vi "MotorMoveIRL.vi"(11 "Rbt Cmd":string) -> ()   [LabVIEW 2019]
uses:
  <vilib>/myRIO/Instrument Drivers/Onboard IO/DIO/typedefs/DIO Reference.ctl
  <vilib>/myRIO/Common/Instrument Driver Framework/Utilities/typedefs/myRIO Generic Hardware Reference.ctl
  <vilib>/myRIO/Common/Instrument Driver Framework/Utilities/typedefs/Hardware Version Enum.ctl
  <vilib>/myRIO/Common/Instrument Driver Framework/Utilities/typedefs/myRIO v1.0 Reference.ctl
  <vilib>/myRIO/Common/Instrument Driver Framework/Utilities/typedefs/Generic FPGA Reference.ctl
  <vilib>/myRIO/Common/Instrument Driver Framework/myRIO v1.0/DIO/typedefs/DIO Channels List.ctl
  <vilib>/myRIO/Common/Instrument Driver Framework/myRIO v1.0/DIO/typedefs/DIO Channels Enum.ctl
  <vilib>/userDefined/High Color/nirio_resource_hc.ctl
  <vilib>/myRIO/Instrument Drivers/Onboard IO/AO/typedefs/AO Reference.ctl
  <vilib>/myRIO/Common/Instrument Driver Framework/myRIO v1.0/AO/typedefs/AO Channels List.ctl
  <vilib>/myRIO/Common/Instrument Driver Framework/myRIO v1.0/AO/typedefs/AO Channels Enum.ctl
  <vilib>/myRIO/Common/Instrument Driver Framework/Utilities/typedefs/Analog Scaling Constants List.ctl
  <vilib>/myRIO/Common/Instrument Driver Framework/Utilities/typedefs/Analog Scaling Constants.ctl
  <vilib>/myRIO/Common/Instrument Driver Framework/myRIO v1.0/Encoder/typedefs/Encoder Signal Mode.ctl
  <vilib>/myRIO/Instrument Drivers/Onboard IO/Encoder/typedefs/Encoder Reference.ctl
  <vilib>/myRIO/Common/Instrument Driver Framework/myRIO v1.0/Encoder/typedefs/Encoder Channels Enum.ctl
  <vilib>/myRIO/Common/Instrument Driver Framework/myRIO v1.0/Encoder/typedefs/Encoder Configuration v1.0.ctl
  <vilib>/myRIO/Common/Instrument Driver Framework/Utilities/vis/Is FPGA Ref Available.vi
  <vilib>/myRIO/Common/Instrument Driver Framework/myRIO v1.0/DIO/vis/myRIO v1.1 Open DIO.vi
  <vilib>/myRIO/Instrument Drivers/Onboard IO/DIO/vis/Write.vi
  <vilib>/myRIO/Common/Instrument Driver Framework/myRIO v1.0/AO/vis/myRIO v1.1 Open AO.vi
  <vilib>/myRIO/Instrument Drivers/Onboard IO/AO/vis/Write.vi
  <vilib>/myRIO/Common/Instrument Driver Framework/myRIO v1.0/Encoder/vis/myRIO v1.1 Open Encoder.vi
  <vilib>/myRIO/Instrument Drivers/Onboard IO/Encoder/vis/Read.vi
  <vilib>/myRIO/Common/Instrument Driver Framework/Utilities/vis/Validate Channels.vi
  <vilib>/myRIO/Common/Instrument Driver Framework/myRIO v1.0/DIO/vis/myRIO v1.0 Reserve DIO.vi
  <vilib>/myRIO/Common/Instrument Driver Framework/myRIO v1.0/AO/vis/myRIO v1.0 Reserve AO.vi
  <vilib>/myRIO/Common/Instrument Driver Framework/myRIO v1.0/Encoder/vis/myRIO v1.0 Reserve Encoder.vi
  <vilib>/myRIO/Common/Instrument Driver Framework/myRIO v1.0/Resource Manager/vis/myRIO v1.0 Reserve Channel List.vi
  <vilib>/myRIO/Common/Instrument Driver Framework/myRIO v1.0/DIO/vis/myRIO v1.0 Build MUX Configuration DIO.vi
  <vilib>/myRIO/Common/Instrument Driver Framework/myRIO v1.0/AO/vis/myRIO v1.0 Build MUX Configuration AO.vi
  <vilib>/myRIO/Common/Instrument Driver Framework/myRIO v1.0/Encoder/vis/myRIO v1.0 Build MUX Configuration Encoder.vi
  <vilib>/myRIO/Common/Instrument Driver Framework/myRIO v1.0/Resource Manager/vis/myRIO v1.0 Reserve Channel.vi
  <vilib>/myRIO/Common/Instrument Driver Framework/myRIO v1.0/Resource Manager/vis/myRIO v1.0 Unreserve Channel.vi
  <vilib>/myRIO/Common/Instrument Driver Framework/myRIO v1.0/Resource Manager/vis/myRIO v1.0 Create Configuration List.vi
  <vilib>/myRIO/Common/Instrument Driver Framework/myRIO v1.0/Resource Manager/vis/myRIO v1.0 Build Mutex Name.vi
  <vilib>/Utility/VariantDataType/GetNumericInfo.vi
  <vilib>/Utility/error.llb/Error Cluster From Error Code.vi
  <vilib>/myRIO/Common/Instrument Driver Framework/myRIO v1.0/myRIO v1.1 Open.vi
  <vilib>/myRIO/Common/Instrument Driver Framework/Utilities/vis/IO Manager.vi
  <vilib>/myRIO/Common/Instrument Driver Framework/Utilities/vis/Configuration Manager.vi
  <vilib>/myRIO/Common/Instrument Driver Framework/myRIO v1.0/Resource Manager/vis/myRIO v1.0 Configure IO.vi
  <vilib>/myRIO/Common/Instrument Driver Framework/myRIO v1.0/myRIO v1.0 Close.vi
  <vilib>/myRIO/Common/Instrument Driver Framework/myRIO v1.0/DIO/vis/myRIO v1.0 Write DIO.vi
  <vilib>/myRIO/Common/Instrument Driver Framework/myRIO v1.0/AO/vis/myRIO v1.0 Get Scaling Constants AO.vi
  <vilib>/myRIO/Common/Instrument Driver Framework/myRIO v1.0/AO/vis/myRIO v1.0 Write AO.vi
  <vilib>/myRIO/Common/Instrument Driver Framework/myRIO v1.0/Encoder/vis/myRIO v1.0 Configure Encoder.vi
  <vilib>/myRIO/Common/Instrument Driver Framework/myRIO v1.0/Encoder/vis/myRIO v1.0 Read Encoder.vi
  <vilib>/myRIO/Express VI/Onboard IO/DO/DO Express VI.xnode
  <vilib>/myRIO/Instrument Drivers/Onboard IO/DIO/vis/myRIO DIO Open.xnode
  <vilib>/myRIO/Express VI/Onboard IO/AO/AO Express VI.xnode
  <vilib>/myRIO/Instrument Drivers/Onboard IO/AO/vis/myRIO AO Open.xnode
  <vilib>/myRIO/Express VI/Onboard IO/Encoder/Encoder Express VI.xnode
  <vilib>/myRIO/Instrument Drivers/Onboard IO/Encoder/vis/myRIO Encoder Open.xnode
  <vilib>/myRIO/Common/Instrument Driver Framework/myRIO v1.0/Encoder/typedefs/Encoder Count Direction Enum.ctl
  <vilib>/myRIO/Instrument Drivers/Onboard IO/Encoder/Encoder.lvlib
  <vilib>/myRIO/Instrument Drivers/Onboard IO/DIO/DIO.lvlib
  <vilib>/myRIO/Instrument Drivers/Onboard IO/AO/AO.lvlib
panel:
  out "Enco D":i32
  out "Enco U":i32
  out "Enco B":i32
  out "Enco R (2)":i32
  out "Enco L (1)":i32
  out "Enco F":i32
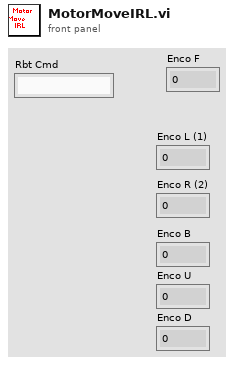
[diagram p1: front panel]
types:
  T1 = typedef "AO.lvlib/AO Reference.ctl" = cluster{"myRIO Reference":T2, "AO Channel List":T6, "AO Scaling Constant List":T8}
  T2 = typedef "myRIO Generic Hardware Reference.ctl" = cluster{"myRIO Model":T3, "myRIO Hardware Reference":T4}
  T3 = typedef "Hardware Version Enum.ctl" = enum16{"Unknown", "myRIO-1900", "myRIO-1950", "roboRIO", "NI ELVIS RIO CM", "ELVIS III"}
  T4 = typedef "myRIO v1.0 Reference.ctl" = cluster{"Generic FPGA Reference":T5, "Allow multiple opens":bool}
  T5 = typedef "Generic FPGA Reference.ctl" = refnum<k20>
  T6 = typedef "AO Channels List.ctl" = T7[]
  T7 = typedef "AO Channels Enum.ctl" = enum16{"Not Connected", "AudioOut/Left", "AudioOut/Right", "C/AO0", "C/AO1", "A/AO0", "A/AO1", "B/AO0", "B/AO1"}
  T8 = typedef "Analog Scaling Constants List.ctl" = T9[]
  T9 = typedef "Analog Scaling Constants.ctl" = cluster{"LSB Weight (Volts)":dbl, "Offset (Volts)":dbl, "Signed?":bool}
  T10 = typedef "nirio_resource_hc.ctl" = tag
  T11 = typedef "Encoder.lvlib/Encoder Reference.ctl" = cluster{"myRIO Reference":T2, "Encoder Channels Enum":T12}
  T12 = typedef "Encoder Channels Enum.ctl" = enum16{"Not Connected", "C/ENC0", "C/ENC1", "A/ENC", "A/ENC0", "A/ENC1", "A/ENC2", "A/ENC3", "A/ENC4", "A/ENC5", "A/ENC6", "A/ENC7", "A/ENC8", "A/ENC9", "B/ENC", "B/ENC0", "B/ENC1", "B/ENC2", "B/ENC3", "B/ENC4", "B/ENC5", "B/ENC6", "B/ENC7", "B/ENC8", "B/ENC9", "DIO/ENC0", "DIO/ENC1", "DIO/ENC2", "DIO/ENC3", "DIO/ENC4"}
  T13 = typedef "Encoder Signal Mode.ctl" = enum16{"Quadrature phase signal", "Step and direction signal"}
  T14 = typedef "DIO.lvlib/DIO Reference.ctl" = cluster{"myRIO Reference":T2, "DIO Channels List":T15}
  T15 = typedef "DIO Channels List.ctl" = T16[]
  T16 = typedef "DIO Channels Enum.ctl" = enum16{"Not Connected", "C/DIO0", "C/DIO1", "C/DIO2", "C/DIO3", "C/DIO4", "C/DIO5", "C/DIO6", "C/DIO7", "A/DIO0", "A/DIO1", "A/DIO2", "A/DIO3", "A/DIO4", "A/DIO5", "A/DIO6", "A/DIO7", "A/DIO8", "A/DIO9", "A/DIO10", "A/DIO11", "A/DIO12", "A/DIO13", "A/DIO14", "A/DIO15", "A/DIO16", "A/DIO17", "A/DIO18", "A/DIO19", "B/DIO0", "B/DIO1", "B/DIO2", "B/DIO3", "B/DIO4", "B/DIO5", "B/DIO6", "B/DIO7", "B/DIO8", "B/DIO9", "B/DIO10", "B/DIO11", "B/DIO12", "B/DIO13", "B/DIO14", "B/DIO15", "B/DIO16", "B/DIO17", "B/DIO18", "B/DIO19", "LED0", "LED1", "LED2", "LED3", "Button0", "DIO/DIO0", "DIO/DIO1", "DIO/DIO2", "DIO/DIO3", "DIO/DIO4", "DIO/DIO5", "DIO/DIO6", "DIO/DIO7", "DIO/DIO8", "DIO/DIO9", "SPI/CS0", "SPI/CS1", "SPI/CS2", "SPI/CS3", "LED RADIO (Green)", "LED RADIO (Red)", "LED COMM (Green)", "LED COMM (Red)", "LED MODE (Green)", "LED MODE (Red)"}
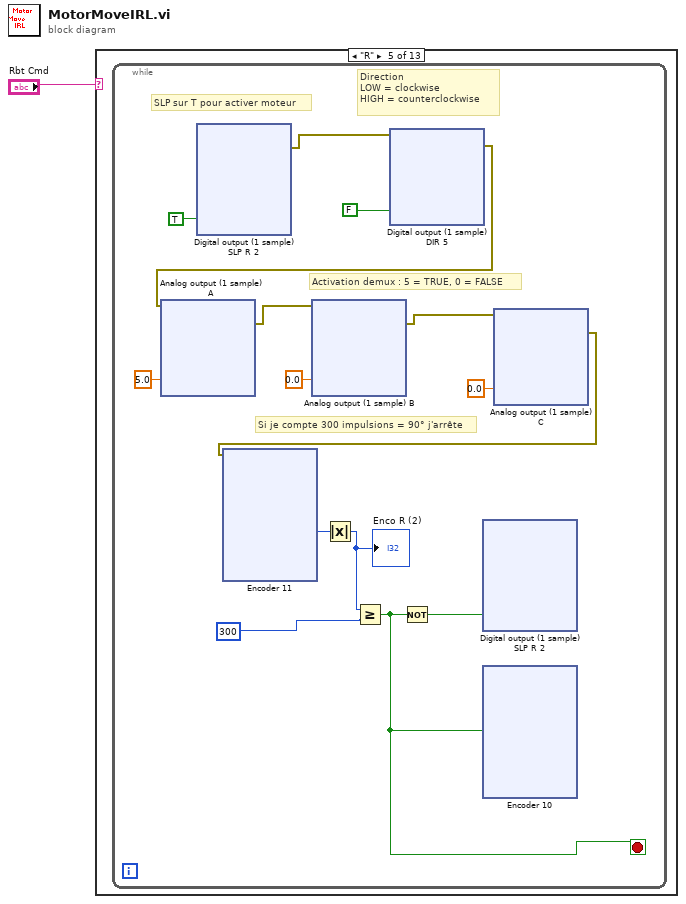
[diagram p0: block diagram]
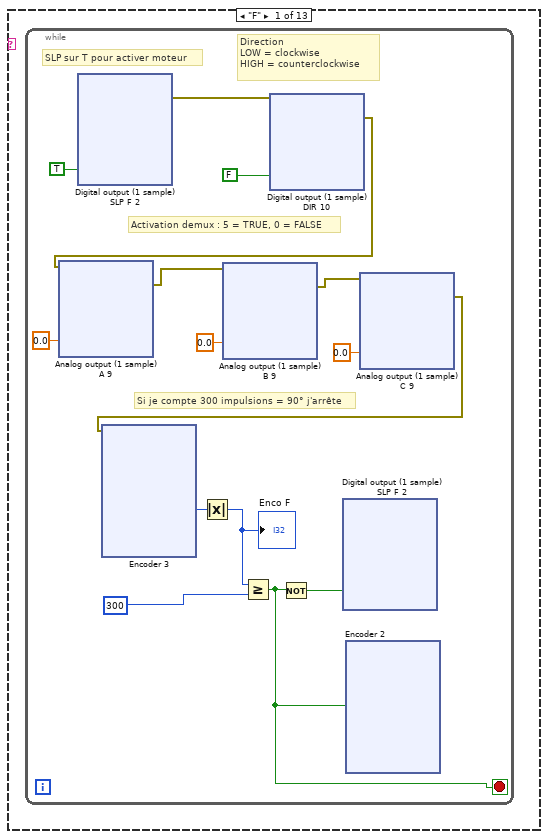
[diagram p2: hidden frame]
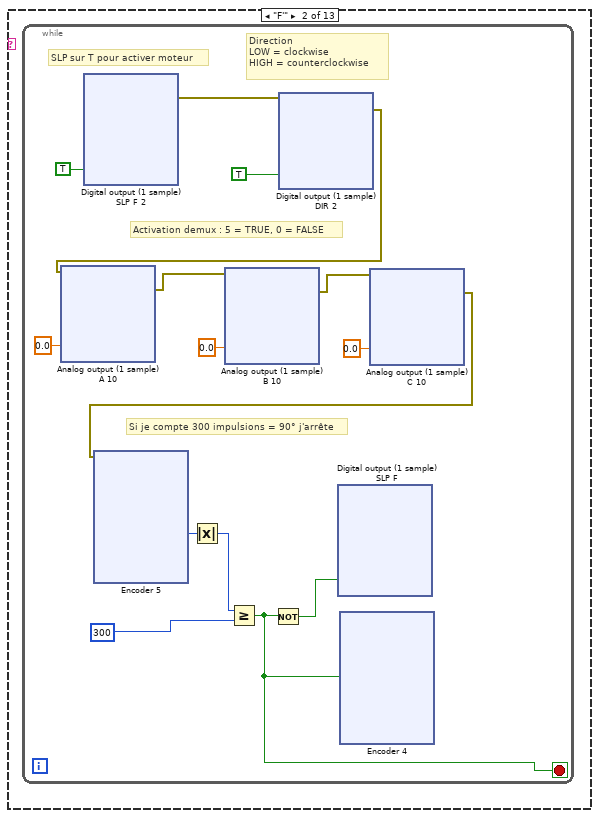
[diagram p3: hidden frame]
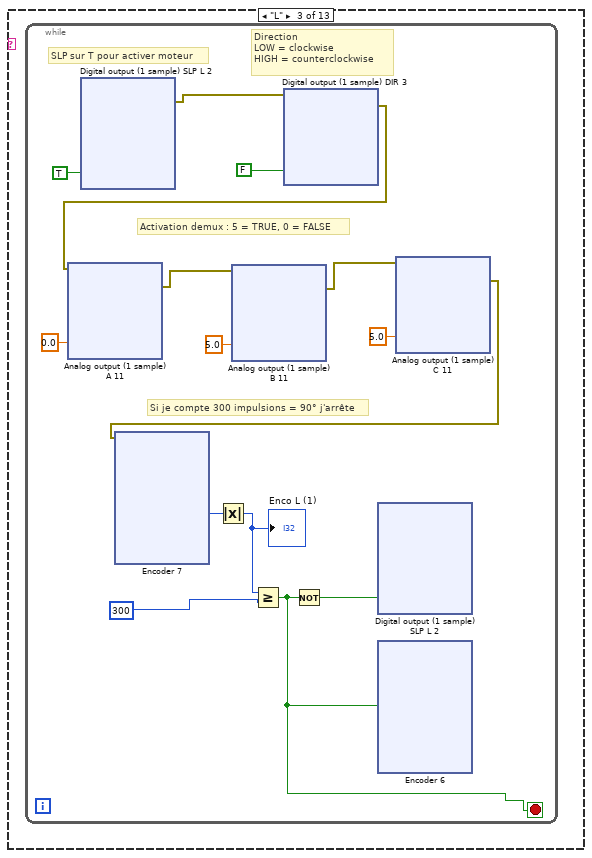
[diagram p4: hidden frame]
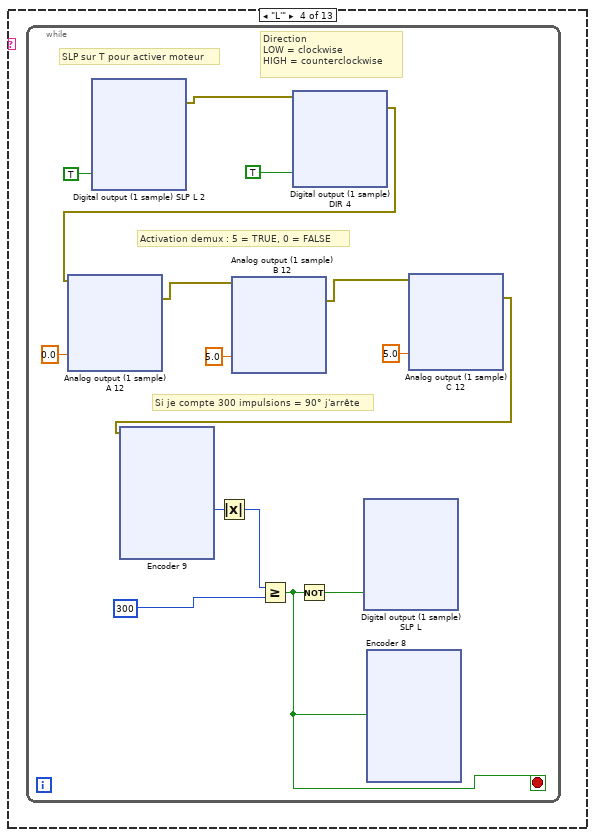
[diagram p5: hidden frame]
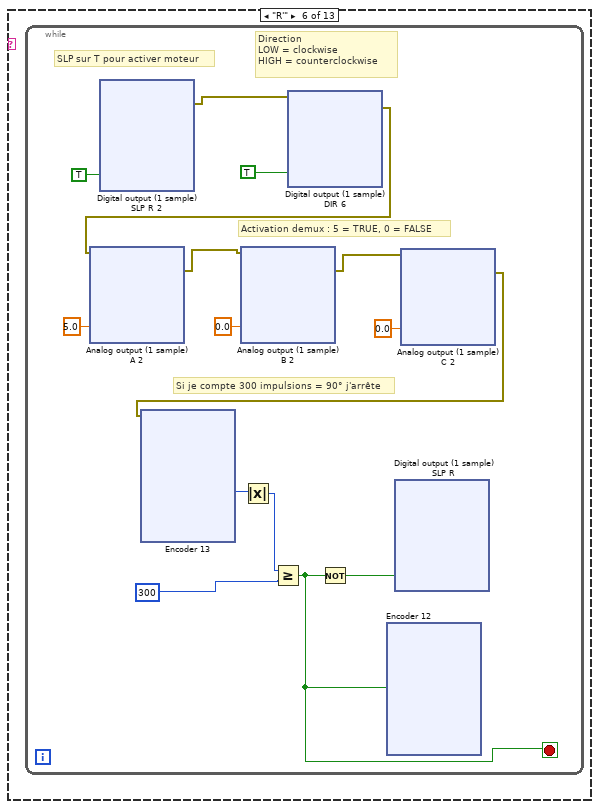
[diagram p6: hidden frame]
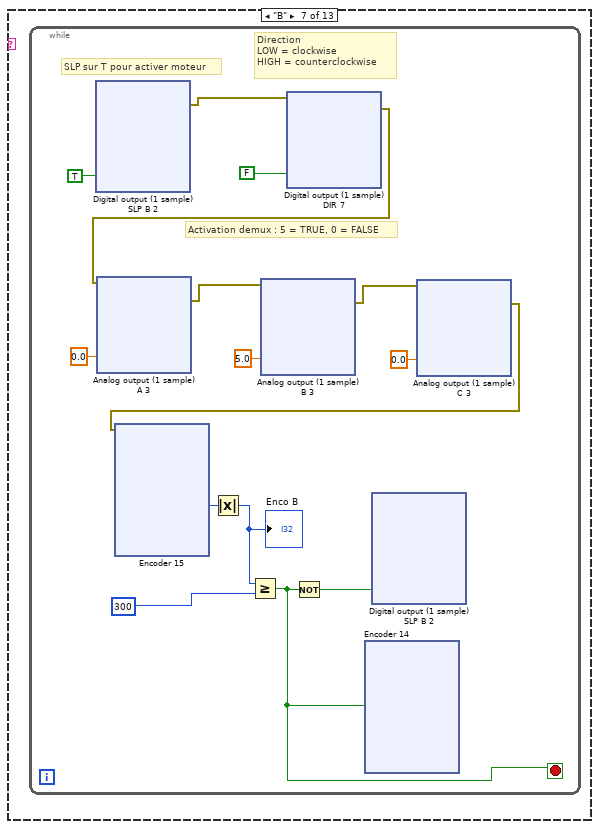
[diagram p7: hidden frame]
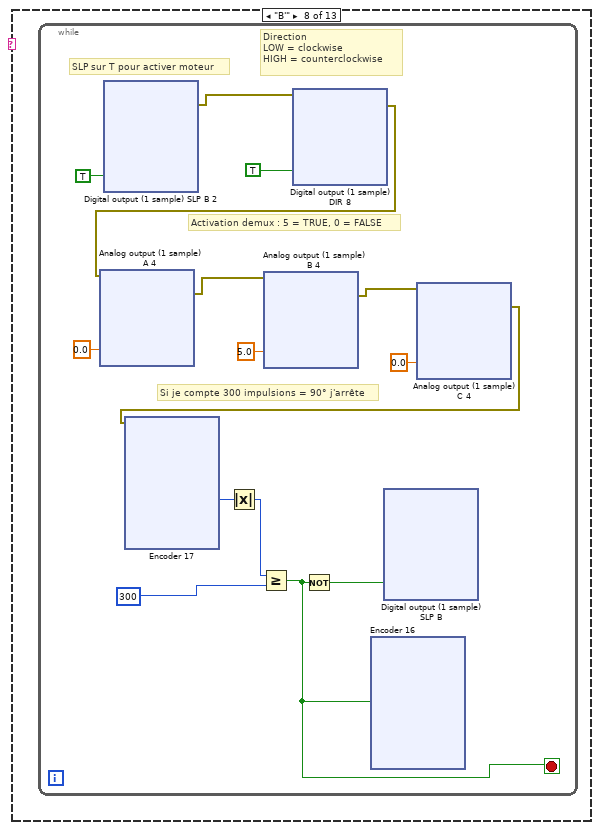
[diagram p8: hidden frame]
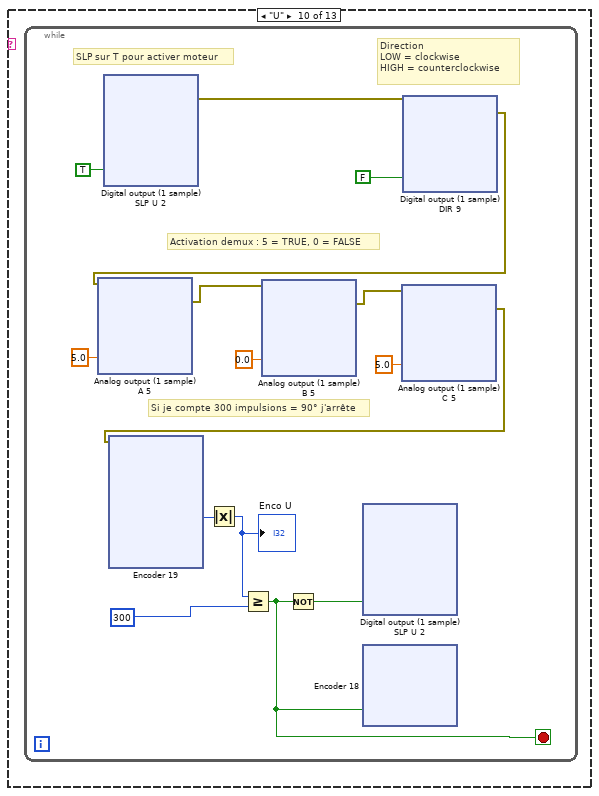
[diagram p10: hidden frame]
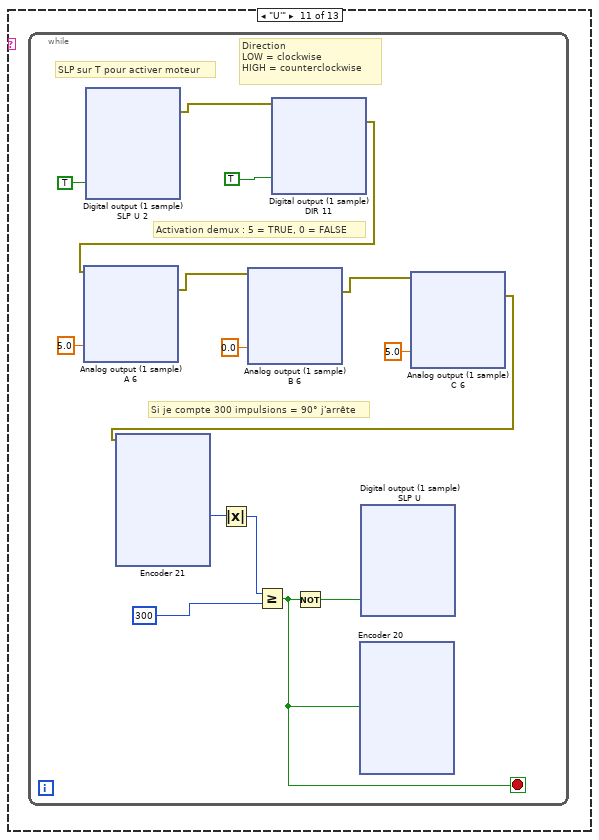
[diagram p11: hidden frame]
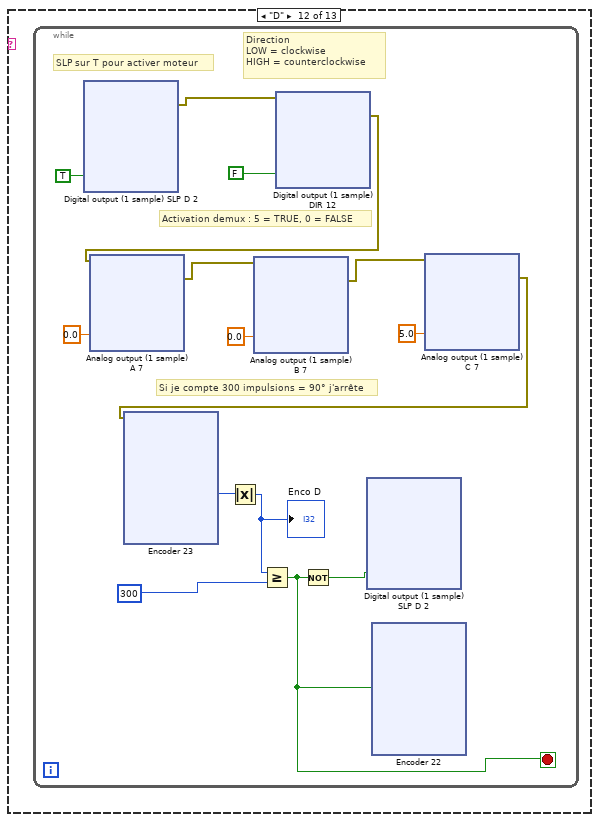
[diagram p12: hidden frame]
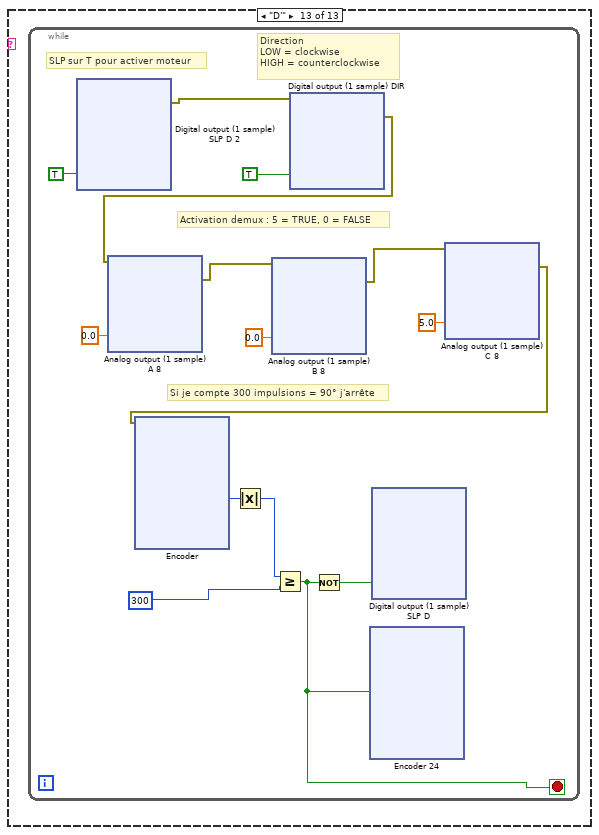
[diagram p13: hidden frame]
diagram:
  n1 = case shown="\"R\"" "Rbt Cmd" {
    frame "F" {
      n2 = while {
        stop <- w10 stop-if-true
        # "Activation demux : 5 = TRUE, 0 = FALSE"
        # "Si je compte 300 impulsions = 90° j'arrête"
        # "SLP sur T pour activer moteur"
        # "Direction\nLOW = clockwise\nHIGH = counterclockwise"
        n3 = xnode "Digital output (1 sample) SLP F 2"("C/DIO0 (DIO0)"=TRUE) -> ("error out"=w6:errorcluster)  [unwired: 1 in]
        n4 = xnode "Digital output (1 sample) DIR 10"("A/DIO0 (Pin 11)"=FALSE, "error in (no error)"=w6) -> ("error out"=w5:errorcluster)
        n5 = xnode "Analog output (1 sample) A 9"("B/AO0 (Pin 2)"=0.0, "error in (no error)"=w5) -> ("error out"=w4:errorcluster)
        n6 = xnode "Analog output (1 sample) B 9"("B/AO1 (Pin 4)"=0.0, "error in (no error)"=w4) -> ("error out"=w3:errorcluster)
        n7 = xnode "Analog output (1 sample) C 9"("A/AO1 (Pin 4)"=0.0 ("C/AO0 (AO0)"), "error in (no error)"=w3) -> ("error out"=w2:errorcluster)
        n8 = xnode "Encoder 3"("error in (no error)"=w2) -> ("Counter Value"=w12:i32)  [unwired: 1 in, 3 out]
        n9 = Absolute Value(x=w12) -> (abs(x)=w13:i32)
        "Enco F" <- w13
        n10 = Greater Or Equal?(x=w13, y=300) -> (x >= y?=w10:bool)
        n11 = Not(x=w10) -> (.not. x?=w14:bool)
        n12 = xnode "Digital output (1 sample) SLP F 2"("C/DIO0 (DIO0)"=w14) -> ()  [unwired: 1 in, 1 out]
        n13 = xnode "Encoder 2"("Reset Counter"=w10) -> ()  [unwired: 1 in, 4 out]
      }
    }
    frame "F'" {
      n14 = while {
        stop <- w338 stop-if-true
        # "Activation demux : 5 = TRUE, 0 = FALSE"
        # "Si je compte 300 impulsions = 90° j'arrête"
        # "SLP sur T pour activer moteur"
        # "Direction\nLOW = clockwise\nHIGH = counterclockwise"
        n15 = xnode "Digital output (1 sample) SLP F 2"("C/DIO0 (DIO0)"=TRUE) -> ("error out"=w329:errorcluster)  [unwired: 1 in]
        n16 = xnode "Digital output (1 sample) DIR 2"("A/DIO0 (Pin 11)"=TRUE, "error in (no error)"=w329) -> ("error out"=w328:errorcluster)
        n17 = xnode "Analog output (1 sample) A 10"("B/AO0 (Pin 2)"=0.0, "error in (no error)"=w328) -> ("error out"=w327:errorcluster)
        n18 = xnode "Analog output (1 sample) B 10"("B/AO1 (Pin 4)"=0.0, "error in (no error)"=w327) -> ("error out"=w326:errorcluster)
        n19 = xnode "Analog output (1 sample) C 10"("A/AO1 (Pin 4)"=0.0 ("C/AO0 (AO0)"), "error in (no error)"=w326) -> ("error out"=w325:errorcluster)
        n20 = xnode "Encoder 5"("error in (no error)"=w325) -> ("Counter Value"=w335:i32)  [unwired: 1 in, 3 out]
        n21 = Absolute Value(x=w335) -> (abs(x)=w334:i32)
        n22 = Greater Or Equal?(x=w334, y=300) -> (x >= y?=w338:bool)
        n23 = Not(x=w338) -> (.not. x?=w336:bool)
        n24 = xnode "Digital output (1 sample) SLP F"("C/DIO0 (DIO0)"=w336) -> ()  [unwired: 1 in, 1 out]
        n25 = xnode "Encoder 4"("Reset Counter"=w338) -> ()  [unwired: 1 in, 4 out]
      }
    }
    frame "L" {
      n26 = while {
        stop <- w661 stop-if-true
        # "Activation demux : 5 = TRUE, 0 = FALSE"
        # "Si je compte 300 impulsions = 90° j'arrête"
        # "SLP sur T pour activer moteur"
        # "Direction\nLOW = clockwise\nHIGH = counterclockwise"
        n27 = xnode "Digital output (1 sample) SLP L 2"("C/DIO3 (DIO3)"=TRUE ("C/DIO0 (DIO0)")) -> ("error out"=w652:errorcluster)  [unwired: 1 in]
        n28 = xnode "Digital output (1 sample) DIR 3"("A/DIO0 (Pin 11)"=FALSE, "error in (no error)"=w652) -> ("error out"=w651:errorcluster)
        n29 = xnode "Analog output (1 sample) A 11"("B/AO0 (Pin 2)"=0.0, "error in (no error)"=w651) -> ("error out"=w650:errorcluster)
        n30 = xnode "Analog output (1 sample) B 11"("B/AO1 (Pin 4)"=5.0, "error in (no error)"=w650) -> ("error out"=w649:errorcluster)
        n31 = xnode "Analog output (1 sample) C 11"("A/AO1 (Pin 4)"=5.0 ("C/AO0 (AO0)"), "error in (no error)"=w649) -> ("error out"=w648:errorcluster)
        n32 = xnode "Encoder 7"("error in (no error)"=w648) -> ("Counter Value"=w658:i32)  [unwired: 1 in, 3 out]
        n33 = Absolute Value(x=w658) -> (abs(x)=w657:i32)
        "Enco L (1)" <- w657
        n34 = Greater Or Equal?(x=w657, y=300) -> (x >= y?=w661:bool)
        n35 = Not(x=w661) -> (.not. x?=w659:bool)
        n36 = xnode "Digital output (1 sample) SLP L 2"("C/DIO3 (DIO3)"=w659) -> ()  [unwired: 1 in, 1 out]
        n37 = xnode "Encoder 6"("Reset Counter"=w661) -> ()  [unwired: 1 in, 4 out]
      }
    }
    frame "L'" {
      n38 = while {
        stop <- w984 stop-if-true
        # "Activation demux : 5 = TRUE, 0 = FALSE"
        # "Si je compte 300 impulsions = 90° j'arrête"
        # "SLP sur T pour activer moteur"
        # "Direction\nLOW = clockwise\nHIGH = counterclockwise"
        n39 = xnode "Digital output (1 sample) SLP L 2"("C/DIO3 (DIO3)"=TRUE ("C/DIO0 (DIO0)")) -> ("error out"=w975:errorcluster)  [unwired: 1 in]
        n40 = xnode "Digital output (1 sample) DIR 4"("A/DIO0 (Pin 11)"=TRUE, "error in (no error)"=w975) -> ("error out"=w974:errorcluster)
        n41 = xnode "Analog output (1 sample) A 12"("B/AO0 (Pin 2)"=0.0, "error in (no error)"=w974) -> ("error out"=w973:errorcluster)
        n42 = xnode "Analog output (1 sample) B 12"("B/AO1 (Pin 4)"=5.0, "error in (no error)"=w973) -> ("error out"=w972:errorcluster)
        n43 = xnode "Analog output (1 sample) C 12"("A/AO1 (Pin 4)"=5.0 ("C/AO0 (AO0)"), "error in (no error)"=w972) -> ("error out"=w971:errorcluster)
        n44 = xnode "Encoder 9"("error in (no error)"=w971) -> ("Counter Value"=w980:i32)  [unwired: 1 in, 3 out]
        n45 = Absolute Value(x=w980) -> (abs(x)=w981:i32)
        n46 = Greater Or Equal?(x=w981, y=300) -> (x >= y?=w984:bool)
        n47 = Not(x=w984) -> (.not. x?=w982:bool)
        n48 = xnode "Digital output (1 sample) SLP L"("C/DIO3 (DIO3)"=w982) -> ()  [unwired: 1 in, 1 out]
        n49 = xnode "Encoder 8"("Reset Counter"=w984) -> ()  [unwired: 1 in, 4 out]
      }
    }
    frame "R" {
      n50 = while {
        stop <- w1307 stop-if-true
        # "Si je compte 300 impulsions = 90° j'arrête"
        # "SLP sur T pour activer moteur"
        # "Activation demux : 5 = TRUE, 0 = FALSE"
        # "Direction\nLOW = clockwise\nHIGH = counterclockwise"
        n51 = xnode "Digital output (1 sample) SLP R 2"("C/DIO1 (DIO1)"=TRUE ("C/DIO0 (DIO0)")) -> ("error out"=w1298:errorcluster)  [unwired: 1 in]
        n52 = xnode "Digital output (1 sample) DIR 5"("A/DIO0 (Pin 11)"=FALSE, "error in (no error)"=w1298) -> ("error out"=w1297:errorcluster)
        n53 = xnode "Analog output (1 sample) A"("B/AO0 (Pin 2)"=5.0, "error in (no error)"=w1297) -> ("error out"=w1296:errorcluster)
        n54 = xnode "Analog output (1 sample) B"("B/AO1 (Pin 4)"=0.0, "error in (no error)"=w1296) -> ("error out"=w1295:errorcluster)
        n55 = xnode "Analog output (1 sample) C"("A/AO1 (Pin 4)"=0.0 ("C/AO0 (AO0)"), "error in (no error)"=w1295) -> ("error out"=w1294:errorcluster)
        n56 = xnode "Encoder 11"("error in (no error)"=w1294) -> ("Counter Value"=w1304:i32)  [unwired: 1 in, 3 out]
        n57 = Absolute Value(x=w1304) -> (abs(x)=w1303:i32)
        "Enco R (2)" <- w1303
        n58 = Greater Or Equal?(x=w1303, y=300) -> (x >= y?=w1307:bool)
        n59 = Not(x=w1307) -> (.not. x?=w1305:bool)
        n60 = xnode "Digital output (1 sample) SLP R 2"("C/DIO1 (DIO1)"=w1305) -> ()  [unwired: 1 in, 1 out]
        n61 = xnode "Encoder 10"("Reset Counter"=w1307) -> ()  [unwired: 1 in, 4 out]
      }
    }
    frame "R'" {
      n62 = while {
        stop <- w1630 stop-if-true
        # "Activation demux : 5 = TRUE, 0 = FALSE"
        # "Si je compte 300 impulsions = 90° j'arrête"
        # "SLP sur T pour activer moteur"
        # "Direction\nLOW = clockwise\nHIGH = counterclockwise"
        n63 = xnode "Digital output (1 sample) SLP R 2"("C/DIO1 (DIO1)"=TRUE ("C/DIO0 (DIO0)")) -> ("error out"=w1621:errorcluster)  [unwired: 1 in]
        n64 = xnode "Digital output (1 sample) DIR 6"("A/DIO0 (Pin 11)"=TRUE, "error in (no error)"=w1621) -> ("error out"=w1620:errorcluster)
        n65 = xnode "Analog output (1 sample) A 2"("B/AO0 (Pin 2)"=5.0, "error in (no error)"=w1620) -> ("error out"=w1619:errorcluster)
        n66 = xnode "Analog output (1 sample) B 2"("B/AO1 (Pin 4)"=0.0, "error in (no error)"=w1619) -> ("error out"=w1618:errorcluster)
        n67 = xnode "Analog output (1 sample) C 2"("A/AO1 (Pin 4)"=0.0 ("C/AO0 (AO0)"), "error in (no error)"=w1618) -> ("error out"=w1617:errorcluster)
        n68 = xnode "Encoder 13"("error in (no error)"=w1617) -> ("Counter Value"=w1627:i32)  [unwired: 1 in, 3 out]
        n69 = Absolute Value(x=w1627) -> (abs(x)=w1626:i32)
        n70 = Greater Or Equal?(x=w1626, y=300) -> (x >= y?=w1630:bool)
        n71 = Not(x=w1630) -> (.not. x?=w1628:bool)
        n72 = xnode "Encoder 12"("Reset Counter"=w1630) -> ()  [unwired: 1 in, 4 out]
        n73 = xnode "Digital output (1 sample) SLP R"("C/DIO1 (DIO1)"=w1628) -> ()  [unwired: 1 in, 1 out]
      }
    }
    frame "B" {
      n74 = while {
        stop <- w1953 stop-if-true
        # "Activation demux : 5 = TRUE, 0 = FALSE"
        # "SLP sur T pour activer moteur"
        # "Direction\nLOW = clockwise\nHIGH = counterclockwise"
        n75 = xnode "Digital output (1 sample) SLP B 2"("C/DIO2 (DIO2)"=TRUE ("C/DIO0 (DIO0)")) -> ("error out"=w1944:errorcluster)  [unwired: 1 in]
        n76 = xnode "Digital output (1 sample) DIR 7"("A/DIO0 (Pin 11)"=FALSE, "error in (no error)"=w1944) -> ("error out"=w1943:errorcluster)
        n77 = xnode "Analog output (1 sample) A 3"("B/AO0 (Pin 2)"=0.0, "error in (no error)"=w1943) -> ("error out"=w1942:errorcluster)
        n78 = xnode "Analog output (1 sample) B 3"("B/AO1 (Pin 4)"=5.0, "error in (no error)"=w1942) -> ("error out"=w1941:errorcluster)
        n79 = xnode "Analog output (1 sample) C 3"("A/AO1 (Pin 4)"=0.0 ("C/AO0 (AO0)"), "error in (no error)"=w1941) -> ("error out"=w1940:errorcluster)
        n80 = xnode "Encoder 15"("error in (no error)"=w1940) -> ("Counter Value"=w1949:i32)  [unwired: 1 in, 3 out]
        n81 = Absolute Value(x=w1949) -> (abs(x)=w1950:i32)
        "Enco B" <- w1950
        n82 = Greater Or Equal?(x=w1950, y=300) -> (x >= y?=w1953:bool)
        n83 = Not(x=w1953) -> (.not. x?=w1951:bool)
        n84 = xnode "Encoder 14"("Reset Counter"=w1953) -> ()  [unwired: 1 in, 4 out]
        n85 = xnode "Digital output (1 sample) SLP B 2"("C/DIO2 (DIO2)"=w1951) -> ()  [unwired: 1 in, 1 out]
      }
    }
    frame "B'" {
      n86 = while {
        stop <- w2276 stop-if-true
        # "Activation demux : 5 = TRUE, 0 = FALSE"
        # "Si je compte 300 impulsions = 90° j'arrête"
        # "SLP sur T pour activer moteur"
        # "Direction\nLOW = clockwise\nHIGH = counterclockwise"
        n87 = xnode "Digital output (1 sample) SLP B 2"("C/DIO2 (DIO2)"=TRUE ("C/DIO0 (DIO0)")) -> ("error out"=w2267:errorcluster)  [unwired: 1 in]
        n88 = xnode "Digital output (1 sample) DIR 8"("A/DIO0 (Pin 11)"=TRUE, "error in (no error)"=w2267) -> ("error out"=w2266:errorcluster)
        n89 = xnode "Analog output (1 sample) A 4"("B/AO0 (Pin 2)"=0.0, "error in (no error)"=w2266) -> ("error out"=w2265:errorcluster)
        n90 = xnode "Analog output (1 sample) B 4"("B/AO1 (Pin 4)"=5.0, "error in (no error)"=w2265) -> ("error out"=w2264:errorcluster)
        n91 = xnode "Analog output (1 sample) C 4"("A/AO1 (Pin 4)"=0.0 ("C/AO0 (AO0)"), "error in (no error)"=w2264) -> ("error out"=w2263:errorcluster)
        n92 = xnode "Encoder 17"("error in (no error)"=w2263) -> ("Counter Value"=w2273:i32)  [unwired: 1 in, 3 out]
        n93 = Absolute Value(x=w2273) -> (abs(x)=w2272:i32)
        n94 = Greater Or Equal?(x=w2272, y=300) -> (x >= y?=w2276:bool)
        n95 = Not(x=w2276) -> (.not. x?=w2274:bool)
        n96 = xnode "Encoder 16"("Reset Counter"=w2276) -> ()  [unwired: 1 in, 4 out]
        n97 = xnode "Digital output (1 sample) SLP B"("C/DIO2 (DIO2)"=w2274) -> ()  [unwired: 1 in, 1 out]
      }
    }
    frame "", Default {
    }
    frame "U" {
      n98 = while {
        stop <- w2599 stop-if-true
        # "Activation demux : 5 = TRUE, 0 = FALSE"
        # "Si je compte 300 impulsions = 90° j'arrête"
        # "SLP sur T pour activer moteur"
        # "Direction\nLOW = clockwise\nHIGH = counterclockwise"
        n99 = xnode "Digital output (1 sample) SLP U 2"("C/DIO5 (DIO5)"=TRUE ("C/DIO0 (DIO0)")) -> ("error out"=w2590:errorcluster)  [unwired: 1 in]
        n100 = xnode "Digital output (1 sample) DIR 9"("A/DIO0 (Pin 11)"=FALSE, "error in (no error)"=w2590) -> ("error out"=w2589:errorcluster)
        n101 = xnode "Analog output (1 sample) A 5"("B/AO0 (Pin 2)"=5.0, "error in (no error)"=w2589) -> ("error out"=w2588:errorcluster)
        n102 = xnode "Analog output (1 sample) B 5"("B/AO1 (Pin 4)"=0.0, "error in (no error)"=w2588) -> ("error out"=w2587:errorcluster)
        n103 = xnode "Analog output (1 sample) C 5"("A/AO1 (Pin 4)"=5.0 ("C/AO0 (AO0)"), "error in (no error)"=w2587) -> ("error out"=w2586:errorcluster)
        n104 = xnode "Encoder 19"("error in (no error)"=w2586) -> ("Counter Value"=w2595:i32)  [unwired: 1 in, 3 out]
        n105 = Absolute Value(x=w2595) -> (abs(x)=w2594:i32)
        "Enco U" <- w2594
        n106 = Greater Or Equal?(x=w2594, y=300) -> (x >= y?=w2599:bool)
        n107 = Not(x=w2599) -> (.not. x?=w2597:bool)
        n108 = xnode "Digital output (1 sample) SLP U 2"("C/DIO5 (DIO5)"=w2597) -> ()  [unwired: 1 in, 1 out]
        n109 = xnode "Encoder 18"("Reset Counter"=w2599) -> ()  [unwired: 1 in, 4 out]
      }
    }
    frame "U'" {
      n110 = while {
        stop <- w2922 stop-if-true
        # "Activation demux : 5 = TRUE, 0 = FALSE"
        # "Si je compte 300 impulsions = 90° j'arrête"
        # "SLP sur T pour activer moteur"
        # "Direction\nLOW = clockwise\nHIGH = counterclockwise"
        n111 = xnode "Digital output (1 sample) SLP U 2"("C/DIO5 (DIO5)"=TRUE ("C/DIO0 (DIO0)")) -> ("error out"=w2913:errorcluster)  [unwired: 1 in]
        n112 = xnode "Digital output (1 sample) DIR 11"("A/DIO0 (Pin 11)"=TRUE, "error in (no error)"=w2913) -> ("error out"=w2912:errorcluster)
        n113 = xnode "Analog output (1 sample) A 6"("B/AO0 (Pin 2)"=5.0, "error in (no error)"=w2912) -> ("error out"=w2911:errorcluster)
        n114 = xnode "Analog output (1 sample) B 6"("B/AO1 (Pin 4)"=0.0, "error in (no error)"=w2911) -> ("error out"=w2910:errorcluster)
        n115 = xnode "Analog output (1 sample) C 6"("A/AO1 (Pin 4)"=5.0 ("C/AO0 (AO0)"), "error in (no error)"=w2910) -> ("error out"=w2909:errorcluster)
        n116 = xnode "Encoder 21"("error in (no error)"=w2909) -> ("Counter Value"=w2917:i32)  [unwired: 1 in, 3 out]
        n117 = Absolute Value(x=w2917) -> (abs(x)=w2918:i32)
        n118 = Greater Or Equal?(x=w2918, y=300) -> (x >= y?=w2922:bool)
        n119 = Not(x=w2922) -> (.not. x?=w2920:bool)
        n120 = xnode "Encoder 20"("Reset Counter"=w2922) -> ()  [unwired: 1 in, 4 out]
        n121 = xnode "Digital output (1 sample) SLP U"("C/DIO5 (DIO5)"=w2920) -> ()  [unwired: 1 in, 1 out]
      }
    }
    frame "D" {
      n122 = while {
        stop <- w3245 stop-if-true
        # "Activation demux : 5 = TRUE, 0 = FALSE"
        # "Si je compte 300 impulsions = 90° j'arrête"
        # "SLP sur T pour activer moteur"
        # "Direction\nLOW = clockwise\nHIGH = counterclockwise"
        n123 = xnode "Digital output (1 sample) SLP D 2"("C/DIO4 (DIO4)"=TRUE ("C/DIO0 (DIO0)")) -> ("error out"=w3236:errorcluster)  [unwired: 1 in]
        n124 = xnode "Digital output (1 sample) DIR 12"("A/DIO0 (Pin 11)"=FALSE, "error in (no error)"=w3236) -> ("error out"=w3235:errorcluster)
        n125 = xnode "Analog output (1 sample) A 7"("B/AO0 (Pin 2)"=0.0, "error in (no error)"=w3235) -> ("error out"=w3234:errorcluster)
        n126 = xnode "Analog output (1 sample) B 7"("B/AO1 (Pin 4)"=0.0, "error in (no error)"=w3234) -> ("error out"=w3233:errorcluster)
        n127 = xnode "Analog output (1 sample) C 7"("A/AO1 (Pin 4)"=5.0 ("C/AO0 (AO0)"), "error in (no error)"=w3233) -> ("error out"=w3232:errorcluster)
        n128 = xnode "Encoder 23"("error in (no error)"=w3232) -> ("Counter Value"=w3242:i32)  [unwired: 1 in, 3 out]
        n129 = Absolute Value(x=w3242) -> (abs(x)=w3241:i32)
        "Enco D" <- w3241
        n130 = Greater Or Equal?(x=w3241, y=300) -> (x >= y?=w3245:bool)
        n131 = Not(x=w3245) -> (.not. x?=w3243:bool)
        n132 = xnode "Digital output (1 sample) SLP D 2"("C/DIO4 (DIO4)"=w3243) -> ()  [unwired: 1 in, 1 out]
        n133 = xnode "Encoder 22"("Reset Counter"=w3245) -> ()  [unwired: 1 in, 4 out]
      }
    }
    frame "D'" {
      n134 = while {
        stop <- w3568 stop-if-true
        # "Activation demux : 5 = TRUE, 0 = FALSE"
        # "Si je compte 300 impulsions = 90° j'arrête"
        # "SLP sur T pour activer moteur"
        # "Direction\nLOW = clockwise\nHIGH = counterclockwise"
        n135 = xnode "Digital output (1 sample) SLP D 2"("C/DIO4 (DIO4)"=TRUE ("C/DIO0 (DIO0)")) -> ("error out"=w3559:errorcluster)  [unwired: 1 in]
        n136 = xnode "Digital output (1 sample) DIR"("A/DIO0 (Pin 11)"=TRUE, "error in (no error)"=w3559) -> ("error out"=w3558:errorcluster)
        n137 = xnode "Analog output (1 sample) A 8"("B/AO0 (Pin 2)"=0.0, "error in (no error)"=w3558) -> ("error out"=w3557:errorcluster)
        n138 = xnode "Analog output (1 sample) B 8"("B/AO1 (Pin 4)"=0.0, "error in (no error)"=w3557) -> ("error out"=w3556:errorcluster)
        n139 = xnode "Analog output (1 sample) C 8"("A/AO1 (Pin 4)"=5.0 ("C/AO0 (AO0)"), "error in (no error)"=w3556) -> ("error out"=w3555:errorcluster)
        n140 = xnode "Encoder"("error in (no error)"=w3555) -> ("Counter Value"=w3565:i32)  [unwired: 1 in, 3 out]
        n141 = Absolute Value(x=w3565) -> (abs(x)=w3564:i32)
        n142 = Greater Or Equal?(x=w3564, y=300) -> (x >= y?=w3568:bool)
        n143 = Not(x=w3568) -> (.not. x?=w3566:bool)
        n144 = xnode "Encoder 24"("Reset Counter"=w3568) -> ()  [unwired: 1 in, 4 out]
        n145 = xnode "Digital output (1 sample) SLP D"("C/DIO4 (DIO4)"=w3566) -> ()  [unwired: 1 in, 1 out]
      }
    }
  }
